vi "Call_Builder_Wiresmith.vi"() -> (2 "Output String":string, 3 "Exit Code":i32)   [LabVIEW 2019]
uses:
  CLI-Inputs.ctl
  TargetType.ctl
  NIPKG Packager/NIPKG Inputs.ctl
  Wiresmith CLI Output/Wiresmith CLI Output.lvclass
  C:/LabVIEW Sources/PPL_Builder/CLI Output/CLI Output.lvclass
  Wiresmith CLI Output/Wiresmith CLI Output.lvclass/Wiresmith CLI Output.ctl
  Builder/Builder.lvclass/Builder.ctl
  Builder/Builder.lvclass
  <vilib>/Wiresmith Technology/G CLI/CLI Class/CLI.lvclass
  NIPKG Packager/NIPKG Packager.lvclass
panel:
  out "CLI Inputs":T1
  out "error out":errorcluster
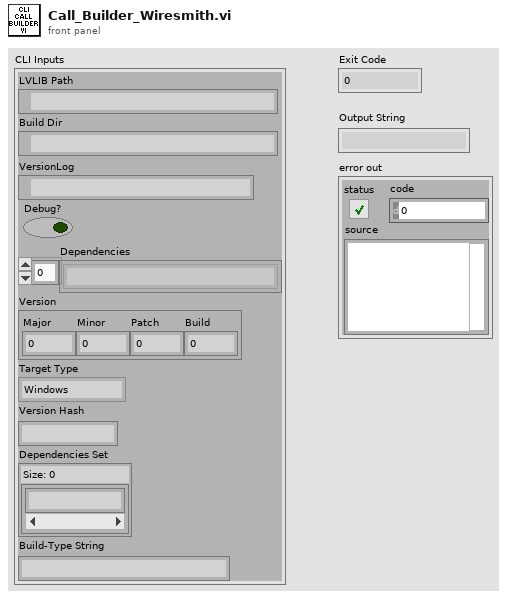
[diagram p1: front panel]
types:
  T1 = typedef "CLI-Inputs.ctl" = cluster{"LVLIB Path":path, "Build Dir":path, "VersionLog":path, "Debug?":bool, "Dependencies":string[], "Version":cluster{"Major":i32, "Minor":i32, "Patch":i32, "Build":i32}, "Target Type":T2, "Version Hash":string, "Dependencies Set":set{string}, "Build Type":string}
  T2 = typedef "TargetType.ctl" = enum16{"Windows", "cRIO-9045"}
  T3 = typedef "NIPKG Packager.lvclass/NIPKG Inputs.ctl" = cluster{"Display Name":string, "Build Type":string, "Version":cluster{"Major":i32, "Minor":i32, "Patch":i32, "Build":i32}, "Dependencies Set":set{string}, "Version Hash":string}
  T4 = cluster{"Major":i32, "Minor":i32, "Patch":i32, "Build":i32}
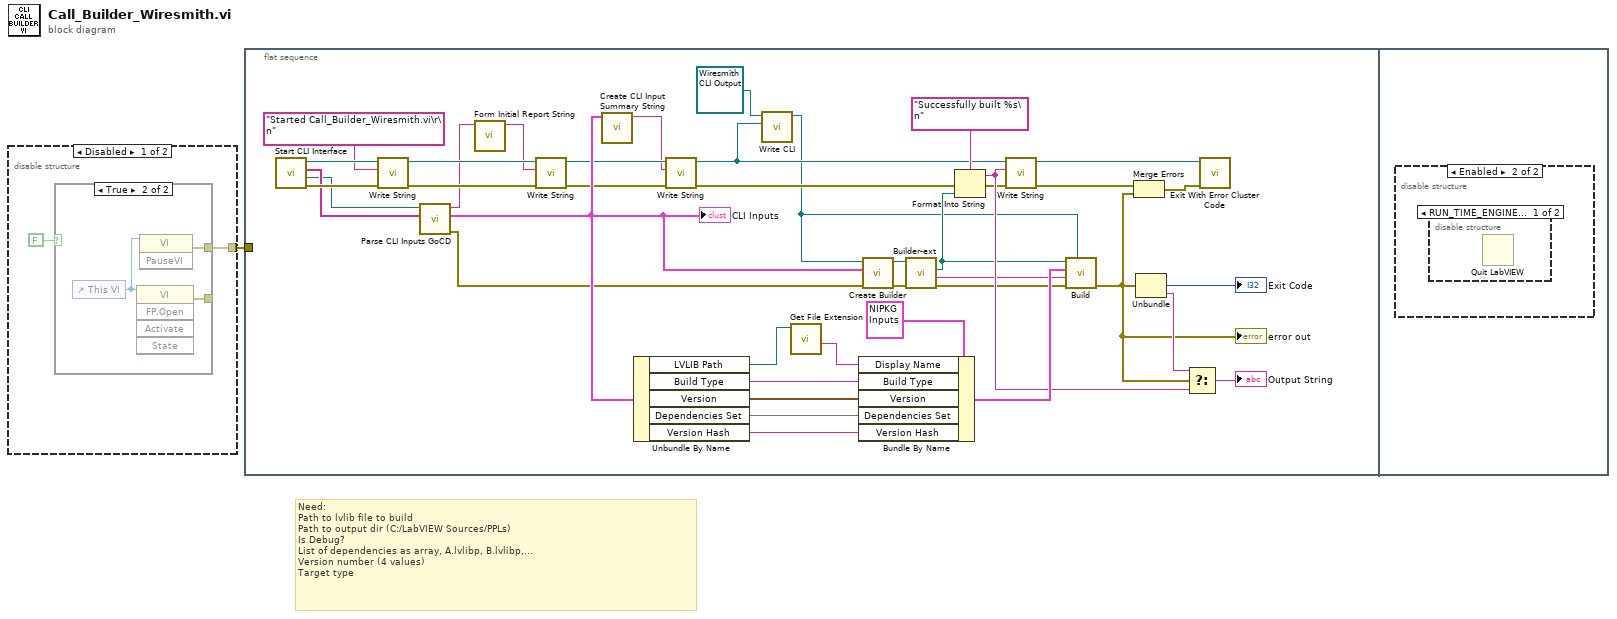
[diagram p0: block diagram]
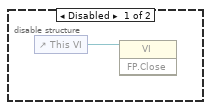
[diagram p2: hidden frame]
diagram:
  # "Need:\nPath to lvlib file to build\nPath to output dir (C:/LabVIEW Sources/PPLs)\nIs Debug?\nList of dependencies as array, A.lvlibp, B.lvlibp,...\nVersion number (4 values)\nTarget type"
  n1 = disable-structure shown="Disabled" {
    disable-tunnel: [w2 _] -> w1
    frame Disabled {
      n2 = case shown="True" FALSE {
        tunnel: [_ w5] -> w2
        tunnel: [_ w4] -> _
        frame False {
        }
        frame True {
          n3 = control-ref of="This VI"() -> (w6:refnum<vi>)
          n4 = invoke class="VI" method="FP.Open"(reference=w6) -> (error out=w4:errorcluster)  [unwired: 4 in, 4 out]
          n5 = invoke class="VI" method="PauseVI"(reference=w6) -> (error out=w5:errorcluster)  [unwired: 2 in, 2 out]
        }
      }
    }
    frame Enabled {
    }
  }
  n6 = flat-sequence {
    tunnel: w1 -> [_]
    frame #0 {
      n7 = call <vilib>:"Start CLI Interface.vi"() -> ("error out"=w12:errorcluster, "Working Directory"=w8:path, "Custom Parameters"=w9:string[], "CLI out"=w11:refnum<class "CLI.lvclass">)  [unwired: 8 in]
      n8 = call <vilib>:"Write String.vi"("error in (no error)"=w12, "Text to Write"="Started Call_Builder_Wiresmith.vi\r\n", "CLI in"=w11) -> ("error out"=w40:errorcluster, "CLI out"=w39:refnum<class "CLI.lvclass">)  [unwired: 7 in]
      n9 = call "Parse CLI Inputs GoCD.vi"("Custom Parameters"=w9, "Working Directory"=w8) -> ("error out"=w36:errorcluster, "CLI Inputs"=w47:T1, "Library Name"=w35:string)  [unwired: 7 in]
      "CLI Inputs" <- w47
      n10 = call "Form Initial Report String.vi"("Library Name"=w35) -> ("String"=w34:string)  [unwired: 10 in]
      n11 = call <vilib>:"Write String.vi"("error in (no error)"=w40, "Text to Write"=w34, "CLI in"=w39) -> ("error out"=w32:errorcluster, "CLI out"=w33:refnum<class "CLI.lvclass">)  [unwired: 7 in]
      n12 = call "Create CLI Input Summary String.vi"("CLI Inputs"=w47) -> ("Summary String"=w31:string)  [unwired: 10 in]
      n13 = Unbundle By Name(w47) -> ("LVLIB Path"=w18:path, "Build Type"=w16:string, "Version"=w15:T4, "Dependencies Set"=w14:set{string}, "Version Hash"=w13:string)
      n14 = call <vilib>:"Write String.vi"("error in (no error)"=w32, "Text to Write"=w31, "CLI in"=w33) -> ("error out"=w26:errorcluster, "CLI out"=w30:refnum<class "CLI.lvclass">)  [unwired: 7 in]
      n15 = call "Write CLI.vi"("CLI"=w30, "Wiresmith CLI Output in"=refnum<class "Wiresmith CLI Output.lvclass"> refnum) -> ("Wiresmith CLI Output out"=w21:refnum<class "Wiresmith CLI Output.lvclass">)  [unwired: 9 in]
      n16 = call <vilib>:"Get File Extension.vi"("file"=w18) -> ("filename without extension"=w17:string)  [unwired: 6 in, 4 out]
      n17 = Bundle By Name(cluster=T3 {"Display Name"="Blah", "Build Type"="cRIO_Debug_32", "Version"={"Major"=0, "Minor"=2, "Patch"=0, "Build"=3}, "Dependencies Set"={}, "Version Hash"="g12421424124"} ("NIPKG Inputs"), "Display Name"=w17, "Build Type"=w16, "Version"=w15, "Dependencies Set"=w14, "Version Hash"=w13) -> (w46:T3)
      n18 = call "Create Builder.vi"("error in (no error)"=w36, "Cluster"=w47, "CLI Output"=w21) -> ("error out"=w37:errorcluster, "Builder out"=w38:refnum<class "Builder.lvclass">)  [unwired: 7 in]
      n19 = call "Builder-ext.vi"("error in (no error)"=w37, "Builder"=w38) -> ("error out"=w24:errorcluster, "Library Description"=w20:string, "Built PPL Path"=w22:path)  [unwired: 7 in]
      n20 = Format Into String(format string="Successfully built %s\n", error in=w26, w22) -> (resulting string=w27:string, error out=w25:errorcluster)  [unwired: 1 in]
      n21 = call <vilib>:"Write String.vi"("error in (no error)"=w25, "Text to Write"=w27, "CLI in"=w30) -> ("error out"=w28:errorcluster, "CLI out"=w29:refnum<class "CLI.lvclass">)  [unwired: 7 in]
      n22 = call "Build.vi"("CLI Output"=w21, "error in (no error)"=w24, "Library Description"=w20, "NIPKG Inputs"=w46, "Installation Path"=w22) -> ("error out"=w23:errorcluster)  [unwired: 6 in]
      "error out" <- w23
      n23 = Merge Errors(w28, w23) -> (w41:errorcluster)
      n24 = Unbundle(w23) -> ("code"=→"Exit Code":i32, "source"=w44:string)  [unwired: 1 out]
      n25 = Select(t=w44, s=w23, f=w27) -> (s? t:f=→"Output String":string)
      n26 = call <vilib>:"Exit With Error Cluster Code.vi"("error in (no error)"=w41, "CLI in"=w29) -> ()  [unwired: 9 in, 1 out]
    }
    frame #1 {
      n27 = disable-structure shown="Enabled" {
        frame Disabled {
          n28 = control-ref of="This VI"() -> (w48:refnum<vi>)
          n29 = invoke class="VI" method="FP.Close"(reference=w48) -> ()  [unwired: 2 in, 3 out]
        }
        frame Enabled {
          n30 = disable-structure shown="RUN_TIME_ENGINE==True" {
            frame condition #0 {
              n31 = Quit LabVIEW() -> ()  [unwired: 1 in]
            }
            frame condition #1 (active) {
            }
          }
        }
      }
    }
  }
